vi "FailResumeMode.vi"(0 "NextMessage":string="5.2.2_Camera Black Level Calibration and Illuminance Verification", 2 "OK/NG":bool, 3 "EndMessage":string="Disconnect_UUT") -> (7 "OutMessage":string)   [LabVIEW 2017]
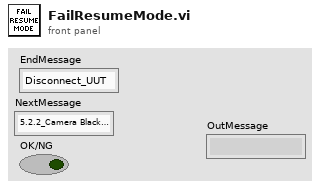
[diagram p1: front panel]
types:
  T1 = typedef "TesterInfo.ctl" = cluster{"Station Name":string, "Station Code":string, "ES NO.":string, "Tester ID":string, "PassMark Revision":string, "Rig ID":string, "682_Tool_Repeat":string, "Project Name":string, "FFTesterPath":path, "Enable_User":bool, "Mode":enum16{"682"}, "Fail_resume_mode":bool}
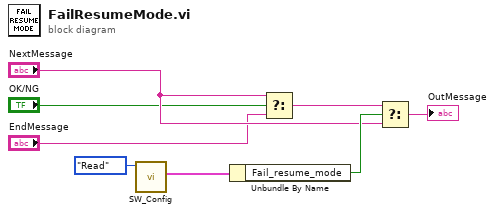
[diagram p0: block diagram]
diagram:
  n1 = call "SW_Config.vi"("Step"=enum16{"Initial", "Write", "Read"}."Read") -> ("SW Config out"=w1:T1)  [unwired: 9 in, 1 out]
  n2 = Unbundle By Name(w1) -> ("Fail_resume_mode"=w8:bool)
  n3 = Select(t="NextMessage", s="OK/NG", f="EndMessage") -> (s? t:f=w5:string)
  n4 = Select(t=w5, s=w8, f="NextMessage") -> (s? t:f=→"OutMessage":string)
